vi "DataSectionCalculator.vi"(2 "Standard Mode #":i8, 3 "CCD ROI":cluster{i32, i32, i32, i32, i32, i32}={0, 4096, 1, 0, 4096, 1}) -> (0 "CCDSUM":string, 1 "TRIMSEC":string)   [LabVIEW 2015]
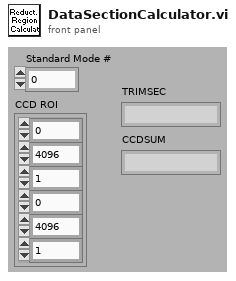
[diagram p1: front panel]
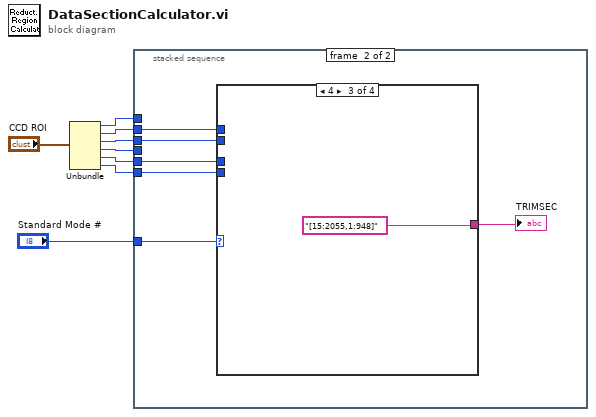
[diagram p0: block diagram]
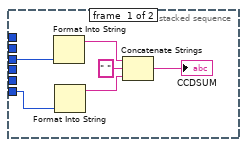
[diagram p2: hidden frame]
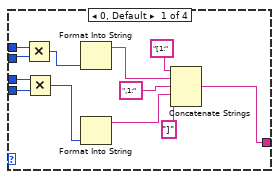
[diagram p3: hidden frame]
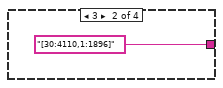
[diagram p4: hidden frame]
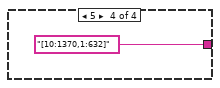
[diagram p5: hidden frame]
diagram:
  n1 = Unbundle("CCD ROI") -> (w7:i32, w6:i32, w5:i32, w4:i32, w3:i32, w2:i32)
  n2 = stacked-sequence {
    tunnel: w7 -> [_ _]
    tunnel: w6 -> [_ w18]
    tunnel: w5 -> [w14 w17]
    tunnel: w4 -> [_ _]
    tunnel: w3 -> [_ w16]
    tunnel: w2 -> [w13 w15]
    tunnel: "Standard Mode #" -> [_ w20]
    frame #0 {
      n3 = Format Into String(w14) -> (resulting string=w12:string)  [unwired: 3 in, 1 out]
      n4 = Format Into String(w13) -> (resulting string=w11:string)  [unwired: 3 in, 1 out]
      n5 = Concatenate Strings(w12, " " ("string"), w11) -> (→"CCDSUM":string)
    }
    frame #1 {
      n6 = case shown="4" w20 {
        tunnel: [w21 "[30:4110,1:1896]" ("TRIMSEC") "[15:2055,1:948]" ("TRIMSEC") "[10:1370,1:632]" ("TRIMSEC")] -> w19
        tunnel: w18 -> [w32 _ _ _]
        tunnel: w17 -> [w31 _ _ _]
        tunnel: w16 -> [w30 _ _ _]
        tunnel: w15 -> [w29 _ _ _]
        frame 0, Default {
          n7 = Multiply(x=w32, y=w31) -> (x*y=w28:i32)
          n8 = Multiply(x=w30, y=w29) -> (x*y=w27:i32)
          n9 = Format Into String(w28) -> (resulting string=w25:string)  [unwired: 3 in, 1 out]
          n10 = Format Into String(w27) -> (resulting string=w23:string)  [unwired: 3 in, 1 out]
          n11 = Concatenate Strings("[1:" ("string"), w25, ",1:" ("string"), w23, "]" ("string")) -> (w21:string)
        }
        frame 3 {
        }
        frame 4 {
        }
        frame 5 {
        }
      }
      "TRIMSEC" <- w19
    }
  }
